vi "OSA_example_analyse.vi"() -> ()   [LabVIEW 2010]
doc: "Single acquisition coherence length example."
uses:
  _OSA_class/typeDef/resolution.ctl
  _OSA_class/typeDef/sensitivityMode.ctl
  _OSA_class/typeDef/interferogram_properties.ctl
  _OSA_class/typeDef/apodisation.ctl
  _OSA_class/typeDef/acq_dataType.ctl
  _misc/Thorlabs_FTS_misc.llb/OSA_virtualModel.ctl
  _misc/Thorlabs_FTS_misc.llb/OSA_virtualSource_RS.ctl
  _misc/Thorlabs_FTS_misc.llb/channelType_spectrum.ctl
  _OSA_class/OSA.lvclass
  OSA20X_misc.lvlib
panel:
  in  "single acq butt":bool
  out "interferogram prop":T1 {"contrast (%)" format="%.2f"; "OPDmax (cm)" format="%.2f"; "OPDmin (cm)" format="%.2f"; "peakToPeak position (cm)" format="%.2f"; "peakToPeak, (counts)" format="%.2f"; "X max (cm)" format="%.2f"; "X min (cm)" format="%.2f"}
  in  "virtual OSA":bool=TRUE
  out "Intensity Graph Interferogram":i32[][](graph)
  in  "spectrIdx":u16
  in  "sensitivity":T2=3 items=["low", "medium", "high"]
  in  "resolution":T3 items=["low", "medium low", "medium high", "high"]
  in  "gain_idx":u16=1
  out "coherence length (cm)":dbl format="%#_6e"
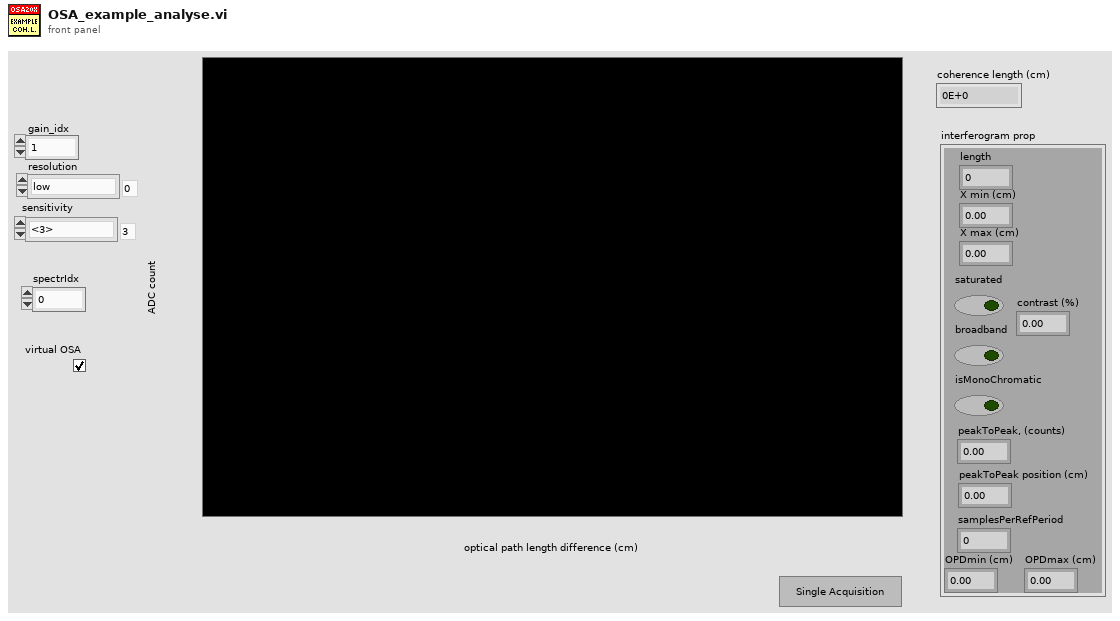
[diagram p1: front panel]
types:
  T1 = typedef "OSA.lvclass/interferogram_properties.ctl" = cluster{"length":u32, "X min (cm)":sgl, "X max (cm)":sgl, "saturated":bool, "broadband":bool, "isMonoChromatic":bool, "peakToPeak, (counts)":dbl, "peakToPeak position (cm)":dbl, "samplesPerRefPeriod":i32, "OPDmin (cm)":sgl, "OPDmax (cm)":sgl, "contrast (%)":dbl}
  T2 = typedef "OSA.lvclass/sensitivityMode.ctl" = u16
  T3 = typedef "OSA.lvclass/resolution.ctl" = u16
  T4 = typedef "OSA20X_misc.lvlib/channelType_spectrum.ctl" = enum16{"SINGLE CHANNEL", "STICHED"}
  T5 = typedef "OSA20X_misc.lvlib/OSA_virtualSource_RS.ctl" = enum16{"VIRTUAL_REDSTONE_SOURCE_UNKNOWN", "VIRTUAL_REDSTONE_SOURCE_LLD_DFB_1530", "VIRTUAL_REDSTONE_SOURCE_SLD_1550nm", "VIRTUAL_REDSTONE_SOURCE_LASER_4600nm", "VIRTUAL_REDSTONE_SOURCE_BLACKBODY1500K", "VIRTUAL_REDSTONE_SOURCE_BLACKBODY1500K_H2O"}
  T6 = cluster{"OSA200":cluster{"waveCenter (nm)":dbl, "FWHM (nm)":dbl, "peakAmplitude":dbl}, "OSA300":T5}
  T7 = typedef "OSA20X_misc.lvlib/OSA_virtualModel.ctl" = enum16{"OSA201", "OSA201C", "OSA202", "OSA202C", "OSA203", "OSA203B", "OSA203C", "OSA205", "OSA205C", "REDSTONE301", "REDSTONE305"}
  T8 = typedef "OSA.lvclass/acq_dataType.ctl" = enum16{"none", "interferogram", "spectrum"}
  T9 = enum16{"full", "zero symmetric (-X min .... +X min)", "zero asymmetric (X min .... X max)"}
  T10 = typedef "OSA.lvclass/apodisation.ctl" = enum16{"NONE", "NORTON_BEER_WEAK", "NORTON_BEER_MEDIUM", "NORTON_BEER_STRONG", "TRIANGULAR", "COSINE", "HANN", "HAMMING", "BLACKMANHARRIS3", "BLACKMANHARRIS4", "GAUSSIAN"}
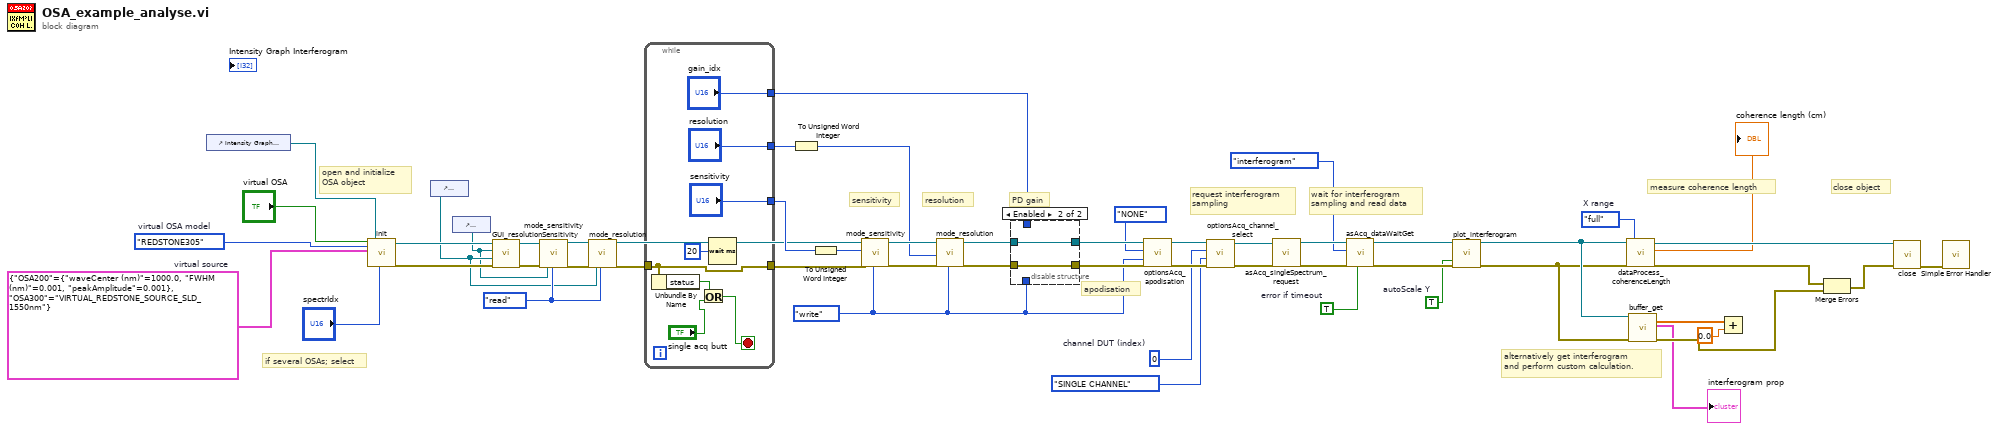
[diagram p0: block diagram]
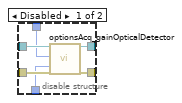
[diagram p2: hidden frame]
diagram:
  w1 = 0  # channel DUT (index)
  w16 = enum16{"read", "write"}."read" ("read/write")
  w22 = T6 {"OSA200"={"waveCenter (nm)"=1000.0, "FWHM (nm)"=0.001, "peakAmplitude"=0.001}, "OSA300"=enum."VIRTUAL_REDSTONE_SOURCE_SLD_1550nm"}  # virtual source
  w23 = OSA_virtualModel."REDSTONE305"  # virtual OSA model
  w29 = TRUE  # autoScale Y
  w35 = TRUE  # error if timeout
  w44 = T9."full"  # X range
  w43 = enum16{"read", "write"}."write" ("read/write")
  # "alternatively get interferogram\nand perform custom calculation."
  # "apodisation"
  # "close object"
  # "open and initialize \nOSA object"
  # "if several OSAs; select"
  # "request interferogram\nsampling"
  # "wait for interferogram \nsampling and read data"
  # "measure coherence length"
  # "PD gain"
  # "resolution"
  # "sensitivity"
  n1 = control-ref of="Intensity Graph Interferogram"() -> (w34:refnum<vi>)
  n2 = call "init.vi"("virtual OSA"="virtual OSA", "virtual OSA model"=w23, "virtual source"=w22, "Graph Intrfrgrm"=w34, "spectrIdx"="spectrIdx") -> ("duplicate reference"=w14:refnum<class "OSA.lvclass">, "error out"=w15:errorcluster)  [unwired: 10 in, 3 out]
  n3 = control-ref of="resolution"() -> (w12:refnum<vi>)
  n4 = control-ref of="sensitivity"() -> (w11:refnum<vi>)
  n5 = call-dynamic "GUI_resolutionSensitivity.vi"("error in (no error)"=w15, "resolution ref"=w12, "sensitivity ref"=w11, "Thorlabs_OSA_64 in"=w14) -> ("error out"=w20:errorcluster, "Thorlabs_OSA_64 out"=w19:refnum<class "OSA.lvclass">)  [unwired: 6 in]
  n6 = call-dynamic "mode_sensitivity.vi"("reference"=w19, "error in (no error)"=w20, "ctrl ref"=w11, "read/write"=w16) -> ("duplicate reference"=w18:refnum<class "OSA.lvclass">, "error out"=w17:errorcluster)  [unwired: 13 in, 1 out]
  n7 = call-dynamic "mode_resolution.vi"("reference"=w18, "error in (no error)"=w17, "ctrl ref"=w12, "read/write"=w16) -> ("duplicate reference"=w13:refnum<class "OSA.lvclass">, "error out"=w8:errorcluster)  [unwired: 12 in, 2 out]
  n8 = while {
    tunnel: ["gain_idx"] -> w47
    tunnel: ["resolution"] -> w46
    tunnel: ["sensitivity"] -> w45
    tunnel: w8 -> [w56]
    tunnel: [w56] -> w7
    stop <- w57 stop-if-true
    n9 = Unbundle By Name(w56) -> ("status"=w58:bool)
    n10 = Or(x=w58, y="single acq butt") -> (x .or. y?=w57:bool)
    n11 = Wait (ms)(milliseconds to wait=u32 20) -> ()  [unwired: 1 out]
  }
  n12 = To Unsigned Word Integer(number=w46) -> (unsigned 16bit integer=w9:T3)
  n13 = To Unsigned Word Integer(number=w45) -> (unsigned 16bit integer=w10:T2)
  n14 = call-dynamic "mode_sensitivity.vi"("reference"=w13, "sensitivity"=w10, "error in (no error)"=w7, "read/write"=w43) -> ("duplicate reference"=w54:refnum<class "OSA.lvclass">, "error out"=w55:errorcluster)  [unwired: 13 in, 1 out]
  n15 = call-dynamic "mode_resolution.vi"("reference"=w54, "resolution"=w9, "error in (no error)"=w55, "read/write"=w43) -> ("duplicate reference"=w52:refnum<class "OSA.lvclass">, "error out"=w53:errorcluster)  [unwired: 12 in, 2 out]
  n16 = disable-structure shown="Enabled" {
    disable-tunnel: w53 -> [w69 w70]
    disable-tunnel: w52 -> [w68 w71]
    disable-tunnel: [w67 w70] -> w50
    disable-tunnel: [w66 w71] -> w49
    disable-tunnel: w47 -> [w65 _]
    disable-tunnel: w43 -> [w64 _]
    frame Disabled {
      n17 = call-dynamic "optionsAcq_gainOpticalDetector.vi"("reference"=w68, "gain_idx"=w65, "readWrite"=w64, "error in (no error)"=w69) -> ("duplicate reference"=w66:refnum<class "OSA.lvclass">, "error out"=w67:errorcluster)  [unwired: 11 in, 3 out]
    }
    frame Enabled {
    }
  }
  n18 = call "optionsAcq_apodisation.vi"("reference"=w49, "apodisation"=apodisation."NONE", "readWrite"=w43, "error in (no error)"=w50) -> ("duplicate reference"=w5:refnum<class "OSA.lvclass">, "error out"=w6:errorcluster)  [unwired: 12 in, 2 out]
  n19 = call-dynamic "optionsAcq_channel_select.vi"("error in (no error)"=w6, "channelType_spectrum"=channelType_spectrum."SINGLE CHANNEL", "channel DUT (index)"=w1, "Thorlabs_OSA_64 in"=w5) -> ("error out"=w3:errorcluster, "Thorlabs_OSA_64 out"=w4:refnum<class "OSA.lvclass">)  [unwired: 5 in, 1 out]
  n20 = call "asAcq_singleSpectrum_request.vi"("reference"=w4, "error in (no error)"=w3) -> ("duplicate reference"=w37:refnum<class "OSA.lvclass">, "error out"=w38:errorcluster)  [unwired: 16 in]
  n21 = call "asAcq_dataWaitGet.vi"("reference"=w37, "dataType"=acq_dataType."interferogram", "error in (no error)"=w38, "error if timeout"=w35) -> ("duplicate reference"=w33:refnum<class "OSA.lvclass">, "error out"=w31:errorcluster)  [unwired: 12 in, 2 out]
  n22 = call "plot_interferogram.vi"("reference"=w33, "autoScale Y"=w29, "error in (no error)"=w31) -> ("duplicate reference"=w32:refnum<class "OSA.lvclass">, "error out"=w30:errorcluster)  [unwired: 15 in]
  n23 = call-dynamic "dataProcess_coherenceLength.vi"("reference"=w32, "error in (no error)"=w30, "X range"=w44) -> ("duplicate reference"=w51:refnum<class "OSA.lvclass">, "coherence length (cm)"=→"coherence length (cm)":dbl, "error out"=w25:errorcluster)  [unwired: 13 in, 1 out]
  n24 = call-dynamic "buffer_get.vi"("reference in"=w32, "error in (no error)"=w30) -> ("interferogram (16bit)"=w41:sgl[], "interferogram prop"=→"interferogram prop":T1, "error out"=w26:errorcluster)  [unwired: 11 in, 4 out]
  n25 = Add(x=w41, y=sgl 0.0 ("Numeric")) -> ()  [unwired: 1 out]
  n26 = Merge Errors(w25, w26) -> (w24:errorcluster)
  n27 = call "close.vi"("reference"=w51, "error in (no error)"=w24) -> ("error out"=w39:errorcluster)  [unwired: 17 in]
  n28 = call <vilib>:"Simple Error Handler.vi"("error in (no error)"=w39) -> ()  [unwired: 4 in, 5 out]
